vi "VDH-calibrateSOLT.vi"(8 "error in (no error)":errorcluster, 10 "VNA data":T2, 11 "VDH-VNA_data_handler in":refnum<class "VDH-VNA_data_handler.lvclass">) -> (0 "error out":errorcluster, 2 "output cluster":T1, 3 "VDH-VNA_data_handler out":refnum<class "VDH-VNA_data_handler.lvclass">)   [LabVIEW 2020, in "VDH-VNA_data_handler.lvlib" / "VDH-VNA_data_handler.lvclass"]
uses:
  VDH-VNA_data_handler.lvclass
  classes/vna-drivers/liteVNA/VD-VNA_data.ctl
  VDH-VNA_data.ctl
  VDH-VNA_data_handler.lvclass/VDH-VNA_data_handler.ctl
  classes/vna-drivers/liteVNA/VD-LV-LiteVNA.lvclass
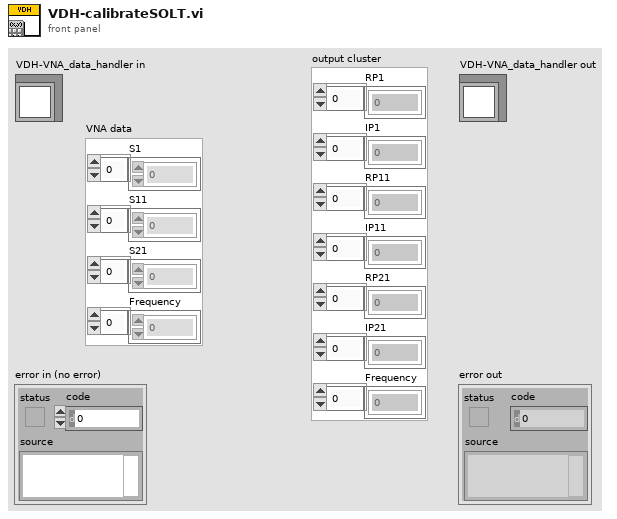
[diagram p1: front panel]
types:
  T1 = typedef "VDH-VNA_data_handler.lvlib/VDH-VNA_data_handler.lvclass/VDH-VNA_data.ctl" = cluster{"RP1":dbl[], "IP1":dbl[], "RP11":dbl[], "IP11":dbl[], "RP21":dbl[], "IP21":dbl[], "Frequency":u64[]}
  T2 = typedef "VD-LV-LiteVNA.lvclass/VD-VNA_data.ctl" = cluster{"S1":cdb[], "S11":cdb[], "S21":cdb[], "Frequency":u64[]}
  T3 = typedef "VDH-VNA_data_handler.lvlib/VDH-VNA_data_handler.lvclass/VDH-Calibration_factor.ctl" = cluster{"A":cdb[], "B":cdb[], "C":cdb[]}
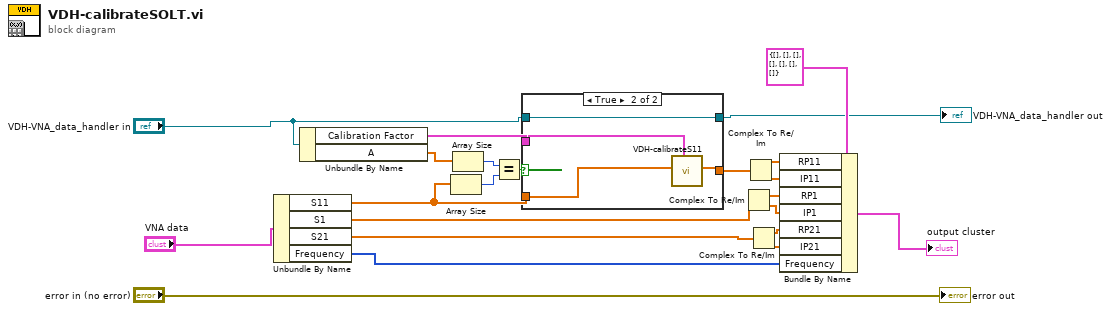
[diagram p0: block diagram]
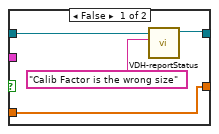
[diagram p2: hidden frame]
diagram:
  n1 = Unbundle By Name("VNA data") -> ("S11"=w8:cdb[], "S1"=w20:cdb[], "S21"=w19:cdb[], "Frequency"=w14:u64[])
  n2 = Unbundle By Name("VDH-VNA_data_handler in") -> ("Calibration Factor"=w9:T3, "A"=w7:cdb[])
  n3 = Array Size(array=w8) -> (size(s)=w5:i32)
  n4 = Array Size(array=w7) -> (size(s)=w6:i32)
  n5 = Equal?(x=w6, y=w5) -> (x = y?=w4:bool)
  n6 = case shown="True" w4 {
    tunnel: [w26 w30] -> w12
    tunnel: w9 -> [_ w29]
    tunnel: w8 -> [w26 w28]
    tunnel: "VDH-VNA_data_handler in" -> [w25 w27]
    tunnel: [w24 w27] -> w2
    frame False {
      n7 = call "VDH-reportStatus.vi"("message"="Calib Factor is the wrong size", "VDH-VNA_data_handler in"=w25) -> ("VDH-VNA_data_handler out"=w24:refnum<class "VDH-VNA_data_handler.lvclass">)  [unwired: 8 in, 1 out]
    }
    frame True {
      n8 = call "VDH-calibrateS11.vi"("Calibration Factor"=w29, "S11"=w28) -> ("S11 out"=w30:cdb[])  [unwired: 9 in]
    }
  }
  "VDH-VNA_data_handler out" <- w2
  n9 = Complex To Re/Im(x + iy=w20) -> (x=w18:dbl[], y=w17:dbl[])
  n10 = Complex To Re/Im(x + iy=w12) -> (x=w11:dbl[], y=w10:dbl[])
  n11 = Complex To Re/Im(x + iy=w19) -> (x=w16:dbl[], y=w15:dbl[])
  n12 = Bundle By Name(cluster=T1 {"RP1"=[], "IP1"=[], "RP11"=[], "IP11"=[], "RP21"=[], "IP21"=[], "Frequency"=[]} ("Data"), "RP11"=w11, "IP11"=w10, "RP1"=w18, "IP1"=w17, "RP21"=w16, "IP21"=w15, "Frequency"=w14) -> (→"output cluster":T1)
  "error out" <- "error in (no error)"
